vi "OAT Waterfall Max Z Range.vi"(6 "zoom factor":i32=5, 8 "spectral map in":dbl[][](array[numeric]) format="%.2f", 9 "Y axis offset":i32=40, 10 "plot settings":T1={"plot color"=0, "grid color"=0, "X shift (rel to total X)"=0.1, "max Z range"=11, "number of spectra"=40} {"max Z range" items=["10^-7", "10^-6", "10^-5", "0.0001", "0.001", "0.01", "0.1", "1", "10", "100", "1000", "auto z range"]; "X shift (rel to total X)" format="%.2f"}, 11 "scale in":cluster{"offset":dbl, "multiplier":dbl} {"multiplier" format="%.2f"; "offset" format="%.2f"}) -> (0 "spectral map out":dbl[][](array[numeric]) format="%.2f", 1 "Y range":cluster{"min":dbl, "max":dbl}={"min"=5.0, "max"=5.0} {"max" format="%.6f"; "min" format="%.6f"}, 2 "plot settings":T1={"plot color"=0, "grid color"=0, "X shift (rel to total X)"=0.1, "max Z range"=11, "number of spectra"=40} {"max Z range" items=["10^-7", "10^-6", "10^-5", "0.0001", "0.001", "0.01", "0.1", "1", "10", "100", "1000", "auto z range"]; "X shift (rel to total X)" format="%.2f"}, 3 "scale out":cluster{"offset":dbl, "multiplier":dbl} {"multiplier" format="%.2f"; "offset" format="%.2f"}, 4 "max Z range":dbl=5.0 format="%.2e")   [LabVIEW 2017]
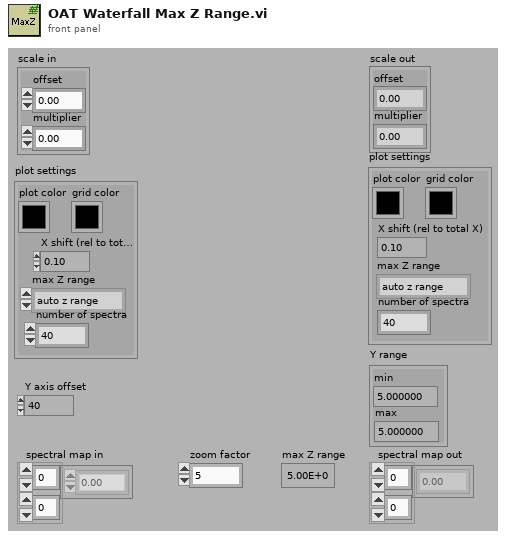
[diagram p1: front panel]
types:
  T1 = cluster{"plot color":u32, "grid color":u32, "X shift (rel to total X)":dbl, "max Z range":u16, "number of spectra":i32}
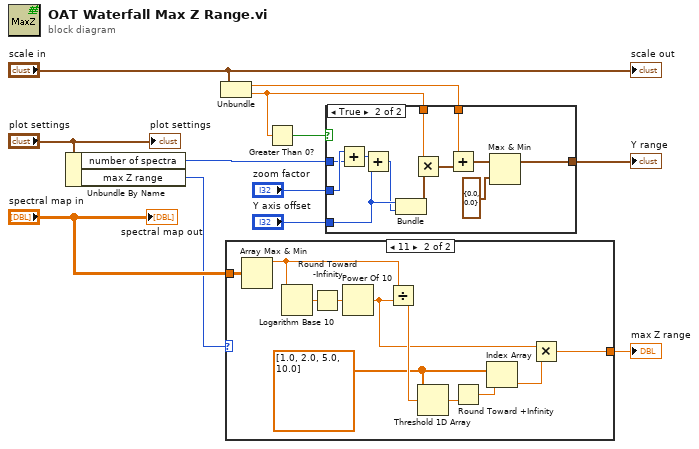
[diagram p0: block diagram]
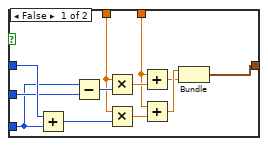
[diagram p2: hidden frame]
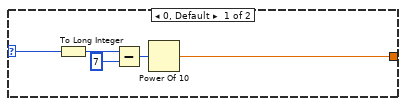
[diagram p3: hidden frame]
diagram:
  n1 = Unbundle By Name("plot settings") -> ("number of spectra"=w5:i32, "max Z range"=w7:u16)
  n2 = Unbundle("scale in") -> ("offset"=w9:dbl, "multiplier"=w3:dbl)
  n3 = case shown="11" w7 {
    selector: w7 -> [w13 _]
    tunnel: [w14 w18] -> w12
    tunnel: "spectral map in" -> [_ w28]
    frame 0, Default {
      n4 = To Long Integer(number=w13) -> (32bit integer=w16:i32)
      n5 = Subtract(x=w16, y=7) -> (x-y=w15:i32)
      n6 = Power Of 10(x=w15) -> (10^x=w14:dbl)
    }
    frame 11 {
      w21 = dbl[] [1.0, 2.0, 5.0, 10.0]
      n7 = Array Max & Min(array=w28) -> (max value=w25:dbl)  [unwired: 3 out]
      n8 = Logarithm Base 10(1:w25) -> (0:w27:dbl)
      n9 = Round Toward -Infinity(1:w27) -> (0:w26:dbl)
      n10 = Power Of 10(x=w26) -> (10^x=w19:dbl)
      n11 = Divide(x=w25, y=w19) -> (x/y=w24:dbl)
      n12 = Threshold 1D Array(2:w24, 3:w21) -> (0:w23:dbl)  [unwired: 1 in]
      n13 = Round Toward +Infinity(x=w23) -> (ceil(x): smallest int >= x=w22:dbl)
      n14 = Index Array(array=w21, index=w22) -> (element=w20:dbl)
      n15 = Multiply(x=w19, y=w20) -> (x*y=w18:dbl)
    }
  }
  "max Z range" <- w12
  n16 = Greater Than 0?(x=w3) -> (x > 0?=w2:bool)
  n17 = case shown="True" w2 {
    tunnel: w9 -> [w35 w42]
    tunnel: "Y axis offset" -> [w30 w50]
    tunnel: "zoom factor" -> [w39 w47]
    tunnel: w5 -> [w40 w46]
    tunnel: [w34 w43] -> w4
    tunnel: w3 -> [w29 w41]
    frame False {
      n18 = Add(x=w40, y=w30) -> (x+y=w33:i32)
      n19 = Subtract(x=w30, y=w39) -> (x-y=w38:i32)
      n20 = Multiply(x=w29, y=w38) -> (x*y=w37:dbl)
      n21 = Multiply(x=w29, y=w33) -> (x*y=w36:dbl)
      n22 = Add(x=w35, y=w37) -> (x+y=w31:dbl)
      n23 = Add(x=w35, y=w36) -> (x+y=w32:dbl)
      n24 = Bundle(w32, w31) -> (w34:cluster{dbl, dbl})  [unwired: 1 in]
    }
    frame True {
      n25 = Add(x=w47, y=w46) -> (x+y=w51:i32)
      n26 = Add(x=w51, y=w50) -> (x+y=w49:i32)
      n27 = Bundle("Y axis offset"=w50, w49) -> (w48:cluster{"Y axis offset":i32, i32})  [unwired: 1 in]
      n28 = Multiply(x=w41, y=w48) -> (x*y=w52:cluster{"Y axis offset":dbl, dbl})
      n29 = Add(x=w42, y=w52) -> (x+y=w44:cluster{"Y axis offset":dbl, dbl})
      n30 = Max & Min(x=w44, y=cluster{"Y axis offset":dbl, dbl} {"Y axis offset"=0.0, 0.0}) -> (max(x,y)=w43:cluster{"Y axis offset":dbl, dbl})  [unwired: 1 out]
    }
  }
  "Y range" <- w4
  "scale out" <- "scale in"
  "spectral map out" <- "spectral map in"
  "plot settings" <- "plot settings"
